vi "svl_Waterfall Global.vi"() -> ()   [LabVIEW 2017]
panel:
  in  "axis labels":T1
  in  "frontmost (T)":bool=TRUE
  in  "display  size":cluster{"width":u32, "heigth":u32}={"width"=400, "heigth"=300}
  in  "occurrence":refnum<k4>
  in  "colors":T2={"frame"=16763904, "plot"=52224, "background"=0}
  in  "autoscale (T)":bool=TRUE
  in  "baseline":dbl format="%.2f"
  in  "set baseline (F)":bool
  in  "clear graph before redrawing (F)":bool
  in  "x0 and delta x":cluster{"x0":dbl, "delta x":dbl}={"x0"=0.0, "delta x"=1.0} {"delta x" format="%.2f"; "x0" format="%.2f"}
  in  "y0 and delta y":cluster{"y0":dbl, "delta y":dbl}={"y0"=0.0, "delta y"=1.0} {"delta y" format="%.2f"; "y0" format="%.2f"}
  in  "waterfall data":dbl[][](array[numeric]) format="%.2f"
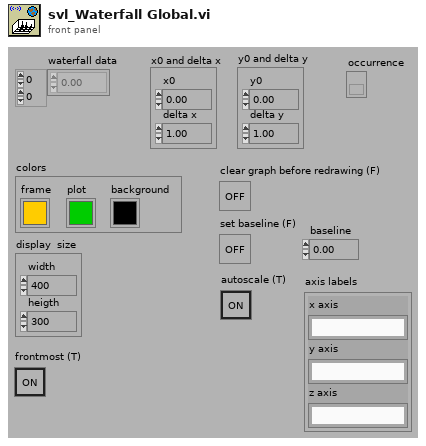
[diagram p1: front panel]
types:
  T1 = cluster{"x axis":string, "y axis":string, "z axis":string}
  T2 = cluster{"frame":u32, "plot":u32, "background":u32}
diagram:
